vi "time_range.vi"(8 "error in (no error)":errorcluster, 10 "Time Range":dbl, 11 "VISA In":refnum<visa-resource-name>) -> (0 "error out":errorcluster, 3 "VISA Out":refnum<visa-resource-name>)   [LabVIEW 2015]
panel:
  out "Sent String":string
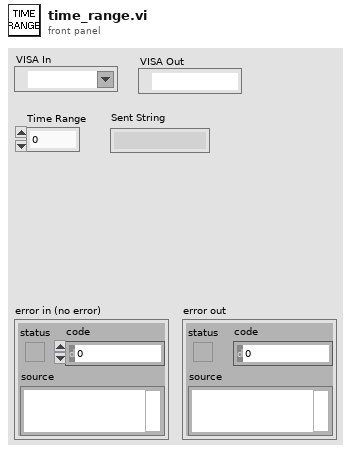
[diagram p1: front panel]
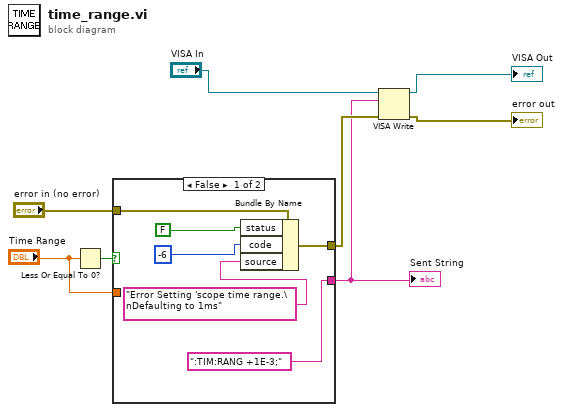
[diagram p0: block diagram]
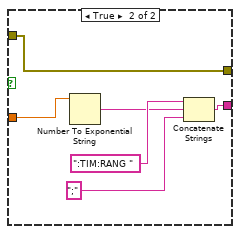
[diagram p2: hidden frame]
diagram:
  n1 = Less Or Equal To 0?(x="Time Range") -> (x <= 0?=w8:bool)
  n2 = case shown="False" w8 {
    tunnel: "Time Range" -> [_ w20]
    tunnel: [":TIM:RANG +1E-3;" w18] -> w1
    tunnel: "error in (no error)" -> [w14 w19]
    tunnel: [w13 w19] -> w4
    frame False {
      n3 = Bundle By Name(cluster=w14, "status"=FALSE, "code"=-6, "source"="Error Setting 'scope time range.\nDefaulting to 1ms") -> (w13:errorcluster)
    }
    frame True {
      n4 = Number To Exponential String(number=w20) -> (E-format string=w16:string)  [unwired: 3 in]
      n5 = Concatenate Strings(":TIM:RANG ", w16, ";") -> (w18:string)
    }
  }
  "Sent String" <- w1
  n6 = VISA Write(VISA resource name="VISA In", write buffer=w1, error in (no error)=w4) -> (VISA resource name out=→"VISA Out":refnum<visa-resource-name>, error out=→"error out":errorcluster)  [unwired: 1 out]
